vi "Read Attribute.vi"(8 "error in (no error)":errorcluster, 11 "Attribute-XML in":refnum<class "Attribute-XML.lvclass">) -> (0 "error out":errorcluster, 2 "Attribute":T1, 3 "Attribute-XML out":refnum<class "Attribute-XML.lvclass">)   [LabVIEW 2013, in "HardwareCharacterization.lvlib" / "Attribute-XML.lvclass"]
uses:
  Attribute-XML.lvclass
  Attributes.ctl
  Attribute-XML.lvclass/Attribute-XML.ctl
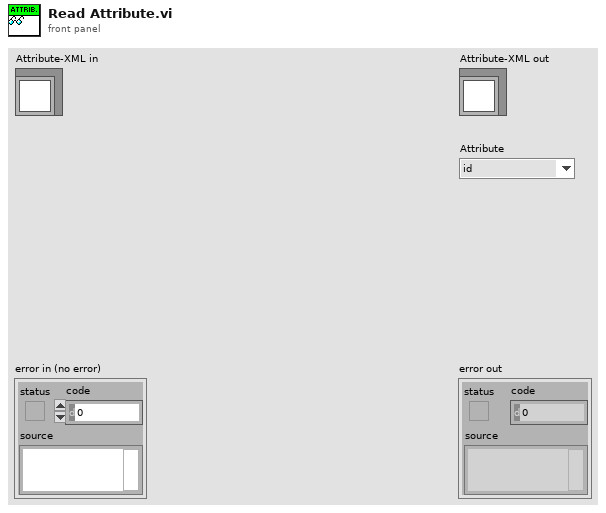
[diagram p1: front panel]
types:
  T1 = typedef "HardwareCharacterization.lvlib/Attribute-XML.lvclass/Attributes.ctl" = enum16{"id"}
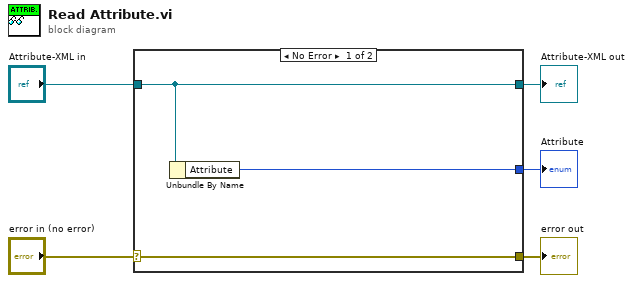
[diagram p0: block diagram]
diagram:
  n1 = case shown="No Error" "error in (no error)" {
    selector: "error in (no error)" -> [w8 w9]
    tunnel: [w8 w9] -> w4
    tunnel: [w7 w10] -> w2
    tunnel: "Attribute-XML in" -> [w7 w10]
    tunnel: [w6 _] -> w1
    frame No Error {
      n2 = Unbundle By Name(w7) -> ("Attribute"=w6:T1)
    }
    frame Error {
    }
  }
  "error out" <- w4
  "Attribute-XML out" <- w2
  "Attribute" <- w1
